vi "movinglog_rangecheck.vi"(1 "naname movingLog(min, max)":i32[][](array[numeric]), 2 "ΔmoveLog(Row, Col.)":i32[][](array[numeric])) -> (0 "daburi":bool)   [LabVIEW 2016]
panel:
  out "範囲内?":bool
  out "i":i32
  out "now_Δ movingLog(min, max)":i32[](array[numeric])
  out "now_naname movingLog(min, max)":i32[](array[numeric])
  out "naname max check":bool
  out "naname min check":bool
  out "Δmin check":bool
  out "Δmax check":bool
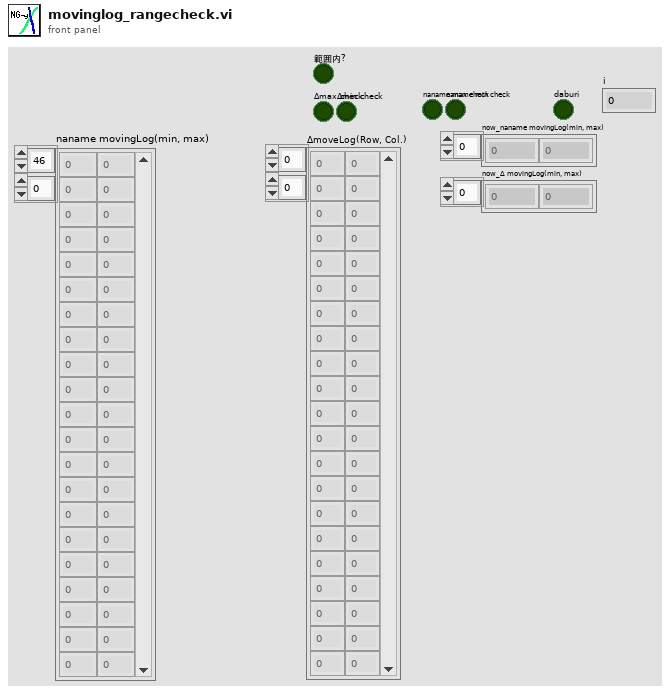
[diagram p1: front panel]
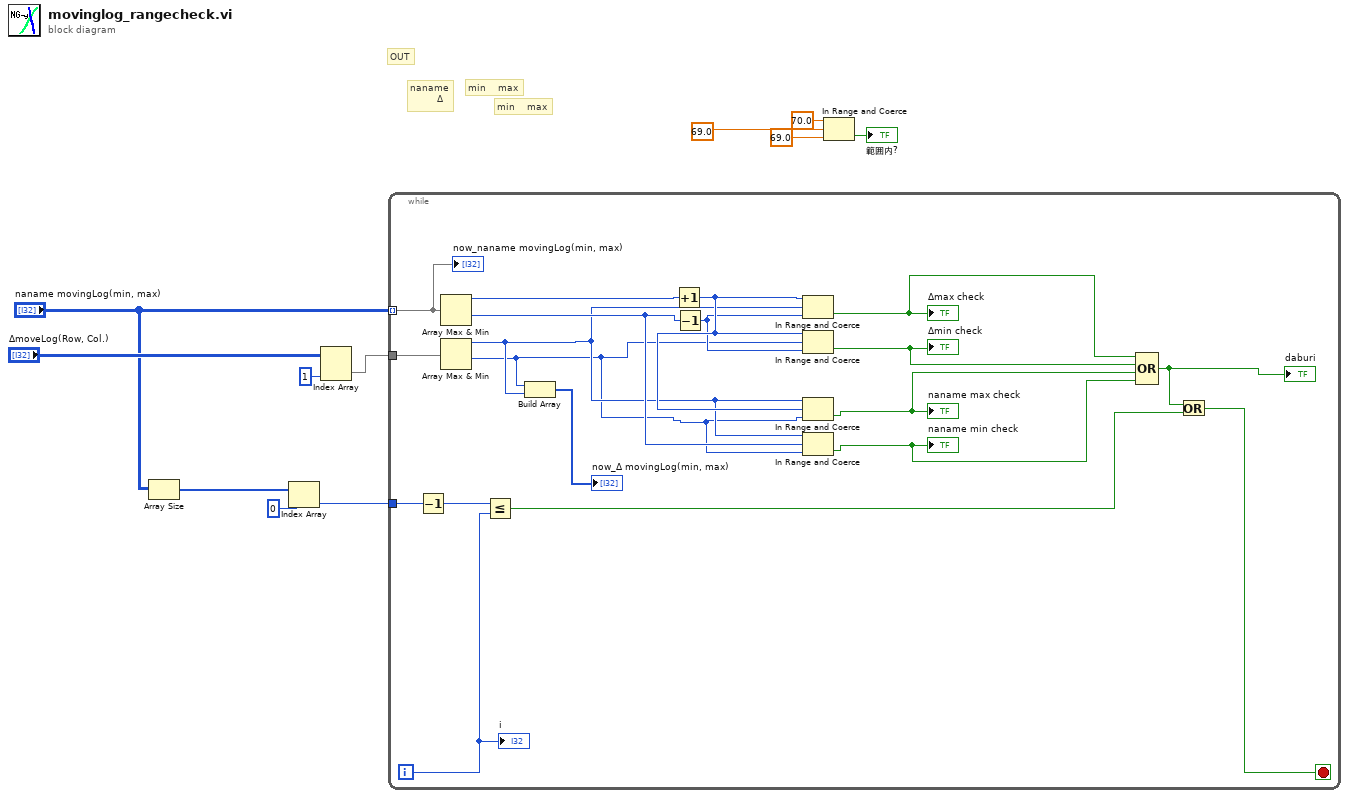
[diagram p0: block diagram]
diagram:
  # "OUT"
  # "min    max"
  # "min    max"
  # "naname\n         Δ"
  n1 = Array Size(array="naname movingLog(min, max)") -> (size(s)=w11:i32[])
  n2 = Index Array(array=w11, index=0 ("指標")) -> (element=w9:i32)
  n3 = Index Array(array="ΔmoveLog(Row, Col.)", index (col)=1 ("無効な指標 （列）")) -> (element=w6:i32[])  [unwired: 1 in]
  n4 = while {
    tunnel: w6 -> [w25]
    tunnel: "naname movingLog(min, max)" -> [w26] mode=indexing
    tunnel: w9 -> [w23]
    i -> [w21]
    stop <- w18 stop-if-true
    n5 = Decrement(x=w23) -> (x-1=w22:i32)
    n6 = Array Max & Min(array=w26) -> (max value=w17:i32, min value=w15:i32)  [unwired: 2 out]
    n7 = Array Max & Min(array=w25) -> (max value=w13:i32, min value=w12:i32)  [unwired: 2 out]
    n8 = Less Or Equal?(x=w22, y=w21) -> (x <= y?=w19:bool)
    n9 = Build Array(w12, w13) -> (→"now_Δ movingLog(min, max)":i32[])
    n10 = Increment(x=w17) -> (x+1=w16:i32)
    n11 = Decrement(x=w15) -> (x-1=w14:i32)
    n12 = In Range and Coerce(upper limit=w16, x=w13, lower limit=w14) -> (In Range?=w30:bool)  [unwired: 1 out]
    "Δmax check" <- w30
    n13 = In Range and Coerce(upper limit=w16, x=w12, lower limit=w14) -> (In Range?=w29:bool)  [unwired: 1 out]
    "Δmin check" <- w29
    n14 = In Range and Coerce(upper limit=w13, x=w16, lower limit=w12) -> (In Range?=w28:bool)  [unwired: 1 out]
    "naname max check" <- w28
    n15 = In Range and Coerce(upper limit=w13, x=w15, lower limit=w12) -> (In Range?=w27:bool)  [unwired: 1 out]
    "naname min check" <- w27
    n16 = Compound Arithmetic op=OR ("複合演算")(w30, w29, w28, w27) -> (w20:bool)
    "daburi" <- w20
    n17 = Or(x=w20, y=w19) -> (x .or. y?=w18:bool)
    "now_naname movingLog(min, max)" <- w26
    "i" <- w21
  }
  n18 = In Range and Coerce(upper limit=70.0 ("上限"), x=69.0, lower limit=69.0 ("下限")) -> (In Range?=→"範囲内?":bool)  [unwired: 1 out]
